vi "Cerebus2LabviewTime.vi"(1 "CerebusTime":string) -> (0 "TimeStamp":timestamp)   [LabVIEW 2011]
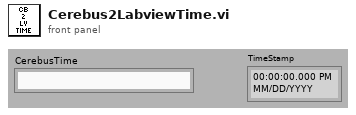
[diagram p1: front panel]
types:
  T1 = cluster{dbl, i32, i32, i32, i32, i32, i32, i32, i32, i32}
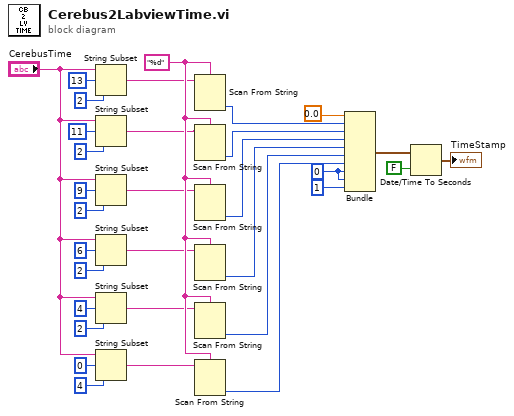
[diagram p0: block diagram]
diagram:
  w31 = 0
  w21 = "%d" ("format string")
  n1 = String Subset(string="CerebusTime", offset (0)=13, length (rest)=2 ("length (rest)")) -> (substring=w15:string)
  n2 = String Subset(string="CerebusTime", offset (0)=11, length (rest)=2 ("length (rest)")) -> (substring=w16:string)
  n3 = String Subset(string="CerebusTime", offset (0)=9, length (rest)=2 ("length (rest)")) -> (substring=w17:string)
  n4 = String Subset(string="CerebusTime", offset (0)=6, length (rest)=2 ("length (rest)")) -> (substring=w18:string)
  n5 = String Subset(string="CerebusTime", offset (0)=4, length (rest)=2 ("length (rest)")) -> (substring=w19:string)
  n6 = String Subset(string="CerebusTime", offset (0)=0, length (rest)=4 ("length (rest)")) -> (substring=w20:string)
  n7 = Scan From String(format string=w21, input string=w15) -> (output 1=w22:i32)  [unwired: 3 in, 3 out]
  n8 = Scan From String(format string=w21, input string=w16) -> (output 1=w23:i32)  [unwired: 3 in, 3 out]
  n9 = Scan From String(format string=w21, input string=w17) -> (output 1=w24:i32)  [unwired: 3 in, 3 out]
  n10 = Scan From String(format string=w21, input string=w18) -> (output 1=w25:i32)  [unwired: 3 in, 3 out]
  n11 = Scan From String(format string=w21, input string=w19) -> (output 1=w26:i32)  [unwired: 3 in, 3 out]
  n12 = Scan From String(format string=w21, input string=w20) -> (output 1=w27:i32)  [unwired: 3 in, 3 out]
  n13 = Bundle(0.0, w22, w23, w24, w25, w26, w27, w31, w31, 1) -> (w30:T1)  [unwired: 1 in]
  n14 = Date/Time To Seconds(1:FALSE ("is UTC (F)"), 2:w30) -> (0:→"TimeStamp":timestamp)
